vi "channel operation tests.vi"() -> ()   [LabVIEW 2013, in "io plugin tests.lvlib"]
uses:
  io plugin tests.lvlib
  module/configuration/tag bus configurable plugin module configuration.lvclass
panel:
  out "error out":errorcluster
  out "channels match":bool
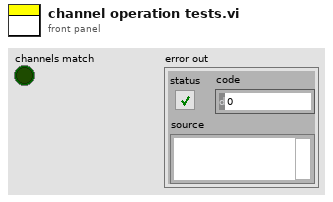
[diagram p1: front panel]
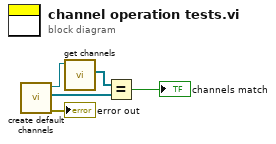
[diagram p0: block diagram]
diagram:
  n1 = call "create default channels.vi"() -> ("error out"=→"error out":errorcluster, "channels"=w1:refnum<class "TBM channel.lvclass">[], "module"=w3:refnum<class "tag bus configurable plugin module configuration.lvclass">)  [unwired: 7 in, 2 out]
  n2 = call-dynamic "get channels.vi"("module configuration in"=w3) -> ("channels"=w5:refnum<class "TBM channel.lvclass">[])  [unwired: 9 in, 1 out]
  n3 = Equal?(x=w5, y=w1) -> (x = y?=→"channels match":bool)
